vi "ClampingTargetDetect.vi"(0 "Image Src":T2) -> (14 "Image Out":T2(plugin-control), 15 "deltax":dbl, 16 "theta":dbl, 17 "distance":dbl, 19 "error out":errorcluster)   [LabVIEW 2011]
uses:
  <vilib>/vision/Image Controls.llb/IMAQ Image.ctl
  <vilib>/vision/Pattern Matching.llb/IMAQ Curve Parameters.ctl
  <vilib>/vision/NI_Vision_Development_Module.lvlib
panel:
  in  "Vertical":T1 {"Rotation" format="%.2f"; "Left" scale=0.0..1024.0; "Right" scale=0.0..1024.0}
  out "deltay":dbl
  in  "d0":dbl=115.0
  in  "p0":dbl=63.0
  in  "thresh":dbl=300.0
  in  "Horizontal":T1 {"Rotation" format="%.2f"; "Left" scale=0.0..1024.0; "Right" scale=0.0..1024.0}
  out "Clamp Points 2":T3
  out "Clamp Points":T3
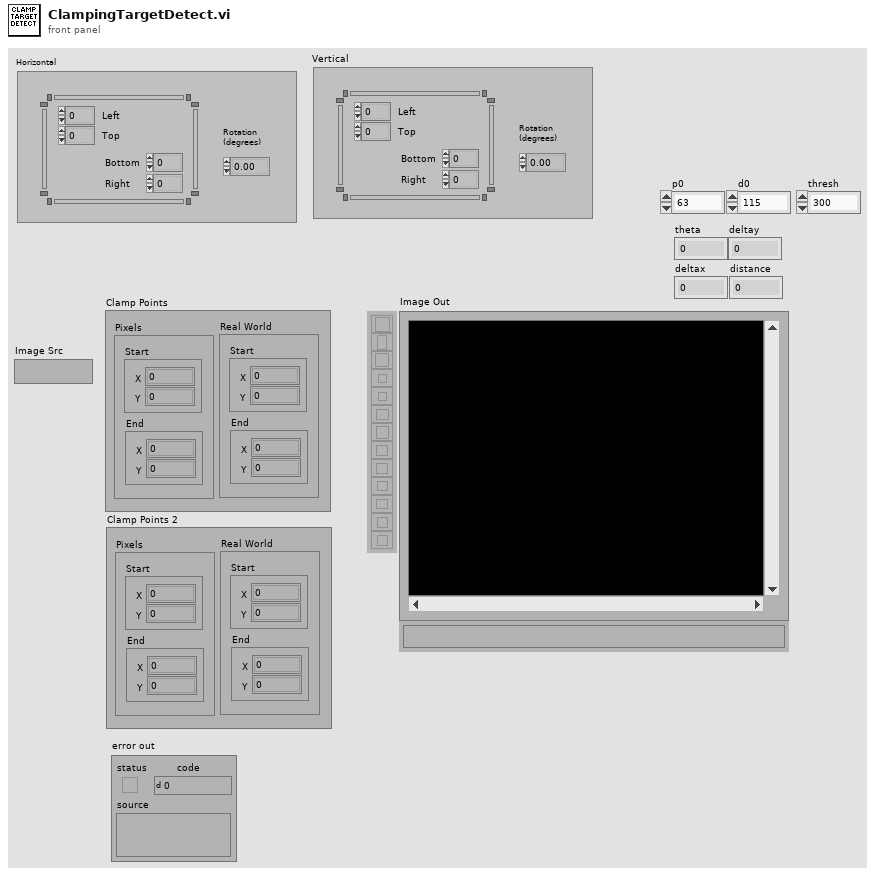
[diagram p1: front panel]
types:
  T1 = typedef "IMAQ Rectangle" = cluster{"Left":i32, "Top":i32, "Right":i32, "Bottom":i32, "Rotation":dbl}
  T2 = typedef "IMAQ Image.ctl" = refnum<image>
  T3 = cluster{"Pixels ":cluster{"Start":cluster{"X":dbl, "Y":dbl}, "End":cluster{"X":dbl, "Y":dbl}}, "Real World":cluster{"Start":cluster{"X":dbl, "Y":dbl}, "End":cluster{"X":dbl, "Y":dbl}}}
  T4 = cluster{"Angle Range (+/-)":dbl, "Edge Polarity":cluster{"Start":u32, "End":u32}}
  T5 = typedef "IMAQ Curve Parameters.ctl" = cluster{"Extraction Mode":u32, "Edge Threshold":i32, "Edge Filter Size":u32, "Min Length":i32, "Row Search Step Size":i32, "Col Search Step Size":i32, "Max Endpoint Gap":i32, "Closed":bool, "Subpixel":bool}
  T6 = cluster{"Show Search Area":bool, "Show Curves":bool, "Show Clamp Locations":bool, "Show Result":bool, "Search Area Color":u32, "Curves Color":u32, "Clamp Locations Color":u32, "Result Color":u32, "Overlay Group Name":string}
  T7 = cluster{"histogram":u32[], "Minimal Value":sgl, "Maximal Value":sgl, "Starting Value":sgl, "Interval Width":sgl, "Mean Value":sgl, "Standard  Variation":sgl, "Area (pixels)":i32}
  T8 = typedef "Image Type" = u32
  T9 = typedef "ROI Descriptor" = cluster{"Global Rectangle":i32[], "Contours":cluster{"ID":enum32{"External", "Internal"}, "Type":u32, "Coordinates":i32[]}[]}
  T10 = cluster{"Distance (Pixels)":dbl, "Distance (Real World)":dbl, "Angle (Absolute)":dbl, "Angle (Relative)":dbl}
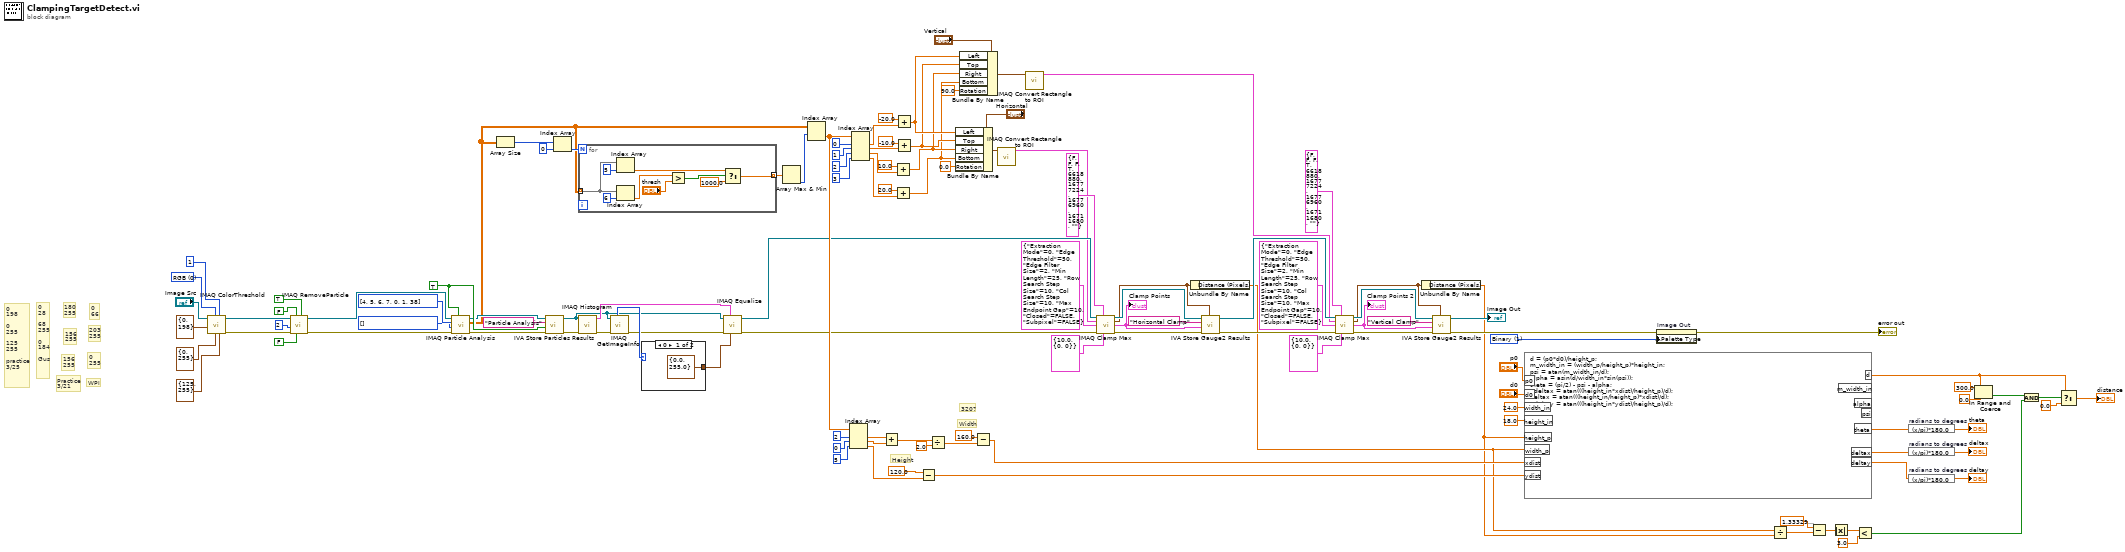
[diagram p0: block diagram]
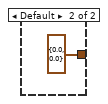
[diagram p2: hidden frame]
diagram:
  w82 = i32[] [] items=["Center of Mass X", "Center of Mass Y", "First Pixel X", "First Pixel Y", "Bounding Rect Left", "Bounding Rect Top", "Bounding Rect Right", "Bounding Rect Bottom", "Max Feret Diameter Start X", "Max Feret Diameter Start Y", "Max Feret Diameter End X", "Max Feret Diameter End Y", "Max Horiz. Segment Length Left", "Max Horiz. Segment Length Right", "Max Horiz. Segment Length Row", "-", "Bounding Rect Width", "Bounding Rect Height", "Bounding Rect Diagonal", "Perimeter", "Convex Hull Perimeter", "Holes' Perimeter", "Max Feret Diameter", "Equivalent Ellipse Major Axis", "Equivalent Ellipse Minor Axis", "Equivalent Ellipse Minor Axis (Feret)", "Equivalent Rect Long Side", "Equivalent Rect Short Side", "Equivalent Rect Diagonal", "Equivalent Rect Short Side (Feret)", "Average Horiz. Segment Length", "Average Vert. Segment Length", "Hydraulic Radius", "Waddel Disk Diameter", "-", "Area", "Holes' Area", "Particle & Holes' Area", "Convex Hull Area", "Image Area", "-", "Number of Holes", "Number of Horiz. Segments", "Number of Vert. Segments", "-", "Orientation", "Max Feret Diameter Orientation", "-", "% Area/Image Area", "% Area/(Particle & Holes' Area)", "Ratio of Equivalent Ellipse Axes", "Ratio of Equivalent Rect Sides", "-", "Elongation Factor", "Compactness Factor", "Heywood Circularity Factor", "Type Factor", "-", "Sum X", "Sum Y", "Sum XX", "Sum XY", "Sum YY", "Sum XXX", "Sum XXY", "Sum XYY", "Sum YYY", "-", "Moment of Inertia XX", "Moment of Inertia XY", "Moment of Inertia YY", "Moment of Inertia XXX", "Moment of Inertia XXY", "Moment of Inertia XYY", "Moment of Inertia YYY", "Norm. Moment of Inertia XX", "Norm. Moment of Inertia XY", "Norm. Moment of Inertia YY", "Norm. Moment of Inertia XXX", "Norm. Moment of Inertia XXY", "Norm. Moment of Inertia XYY", "Norm. Moment of Inertia YYY", "Hu Moment 1", "Hu Moment 2", "Hu Moment 3", "Hu Moment 4", "Hu Moment 5", "Hu Moment 6", "Hu Moment 7"] ("Real-World Measurements")
  w83 = i32[] [4, 5, 6, 7, 0, 1, 38] items=["Center of Mass X", "Center of Mass Y", "First Pixel X", "First Pixel Y", "Bounding Rect Left", "Bounding Rect Top", "Bounding Rect Right", "Bounding Rect Bottom", "Max Feret Diameter Start X", "Max Feret Diameter Start Y", "Max Feret Diameter End X", "Max Feret Diameter End Y", "Max Horiz. Segment Length Left", "Max Horiz. Segment Length Right", "Max Horiz. Segment Length Row", "-", "Bounding Rect Width", "Bounding Rect Height", "Bounding Rect Diagonal", "Perimeter", "Convex Hull Perimeter", "Holes' Perimeter", "Max Feret Diameter", "Equivalent Ellipse Major Axis", "Equivalent Ellipse Minor Axis", "Equivalent Ellipse Minor Axis (Feret)", "Equivalent Rect Long Side", "Equivalent Rect Short Side", "Equivalent Rect Diagonal", "Equivalent Rect Short Side (Feret)", "Average Horiz. Segment Length", "Average Vert. Segment Length", "Hydraulic Radius", "Waddel Disk Diameter", "-", "Area", "Holes' Area", "Particle & Holes' Area", "Convex Hull Area", "Image Area", "-", "Number of Holes", "Number of Horiz. Segments", "Number of Vert. Segments", "-", "Orientation", "Max Feret Diameter Orientation", "-", "% Area/Image Area", "% Area/(Particle & Holes' Area)", "Ratio of Equivalent Ellipse Axes", "Ratio of Equivalent Rect Sides", "-", "Elongation Factor", "Compactness Factor", "Heywood Circularity Factor", "Type Factor", "-", "Sum X", "Sum Y", "Sum XX", "Sum XY", "Sum YY", "Sum XXX", "Sum XXY", "Sum XYY", "Sum YYY", "-", "Moment of Inertia XX", "Moment of Inertia XY", "Moment of Inertia YY", "Moment of Inertia XXX", "Moment of Inertia XXY", "Moment of Inertia XYY", "Moment of Inertia YYY", "Norm. Moment of Inertia XX", "Norm. Moment of Inertia XY", "Norm. Moment of Inertia YY", "Norm. Moment of Inertia XXX", "Norm. Moment of Inertia XXY", "Norm. Moment of Inertia XYY", "Norm. Moment of Inertia YYY", "Hu Moment 1", "Hu Moment 2", "Hu Moment 3", "Hu Moment 4", "Hu Moment 5", "Hu Moment 6", "Hu Moment 7"] ("Pixel Measurements")
  w81 = TRUE ("Connectivity 4/8 (8)")
  w86 = u32 1 items=["Grayscale", "Binary", "Gradient", "Rainbow", "Temperature", "User Defined"] ("Palette")
  w119 = u16 0 items=["RGB", "HSL", "HSV", "HSI"] ("Color Mode")
  # "320?"
  # "0\n198\n\n0\n255\n\n125\n255\n\npractice\n3/25"
  # "0\n28\n\n68\n255\n\n0\n184\n\nGus"
  # "Practice\n3/21"
  # "WPI"
  # "156\n255"
  # "156\n255"
  # "180\n255"
  # "0\n255"
  # "203\n255"
  # "0\n66"
  # "Width"
  # "Height"
  n1 = call "IMAQ ColorThreshold"("Blue or Luma or Val or Inten Range"=cluster{"Lower value":i32, "Upper value":i32} {"Lower value"=125, "Upper value"=255}, "Replace Value"=1, "Green or Sat Range"=cluster{"Lower value":i32, "Upper value":i32} {"Lower value"=0, "Upper value"=255}, "Color Mode"=w119, "Red or Hue Range"=cluster{"Lower value":i32, "Upper value":i32} {"Lower value"=0, "Upper value"=198}, "Image Src"="Image Src") -> ("error out"=w115:errorcluster, "Image Dst Out"=w110:T2)  [unwired: 2 in, 2 out]
  n2 = call "IMAQ RemoveParticle"("Connectivity 4/8 (8)"=TRUE, "Low Pass/High Pass (Low)"=FALSE, "Square/Hexa (Square)"=FALSE, "error in (no error)"=w115, "Number of Erosion"=2, "Image Src"=w110) -> ("error out"=w43:errorcluster, "Image Dst Out"=w44:T2)  [unwired: 1 in, 3 out]
  n3 = call "IMAQ Particle Analysis"("Connectivity 4/8 (8)"=w81, "error in (no error)"=w43, "Real-World Measurements"=w82, "Pixel Measurements"=w83, "Image"=w44) -> ("error out"=w78:errorcluster, "Particle Measurements (Pixels)"=w56:dbl[][], "Image Out (duplicate)"=w80:T2)  [unwired: 4 out]
  n4 = Array Size(array=w56) -> (size(s)=w62:i32[])
  n5 = call <vilib>:"IVA Store Particles Results.vi"("error in (no error)"=w78, "Connectivity 4/8 (8)"=w81, "Step Name"="Particle Analysis", "Image in"=w80) -> ("error out"=w26:errorcluster, "Image dup"=w25:T2)  [unwired: 6 out]
  n6 = Index Array(array=w62, index=0) -> (element=w60:i32)
  n7 = for {
    N: w60 -> [_]
    tunnel: w56 -> [w127] mode=indexing
    tunnel: [w121] -> w55 mode=indexing
    n8 = Index Array(array=w127, index=5) -> (element=w123:dbl)
    n9 = Index Array(array=w127, index=6) -> (element=w126:dbl)
    n10 = Greater?(x=w126, y="thresh") -> (0:w124:bool)
    n11 = Select(t=w123, s=w124, f=1000.0) -> (s? t:f=w121:dbl)
  }
  n12 = call "IMAQ Histogram"("error in (no error)"=w26, "Image"=w25) -> ("error out"=w107:errorcluster, "Histogram Report"=w109:T7)  [unwired: 3 in, 5 out]
  n13 = call "IMAQ GetImageInfo"("error in (no error)"=w107, "Image"=w25) -> ("error out"=w106:errorcluster, "Image Type"=w108:T8)  [unwired: 8 out]
  n14 = case shown="0" w108 {
    tunnel: [cluster{"Minimum":sgl, "Maximum":sgl} {"Minimum"=0.0, "Maximum"=255.0} ("Range") cluster{"Minimum":sgl, "Maximum":sgl} {"Minimum"=0.0, "Maximum"=0.0} ("Range")] -> w105
    frame 0 {
    }
    frame Default {
    }
  }
  n15 = call "IMAQ Equalize"("Range"=w105, "Histogram Report"=w109, "error in (no error)"=w106, "Image Src"=w25) -> ("error out"=w45:errorcluster, "Image Dst Out"=w46:T2)  [unwired: 2 in, 4 out]
  n16 = Array Max & Min(array=w55) -> (min index (indices)=w59:i32)  [unwired: 3 out]
  n17 = Index Array(array=w56, index (row)=w59) -> (element=w65:dbl[])  [unwired: 1 in]
  n18 = Index Array(array=w65, index #1=2 ("index"), index #2=0 ("index"), index #3=5 ("index")) -> (element #1=w52:dbl, element #2=w51:dbl, element #3=w53:dbl)
  n19 = Index Array(array=w65, index #1=0 ("index"), index #2=1 ("index"), index #3=2 ("index"), index #4=3 ("index")) -> (element #1=w67:dbl, element #2=w72:dbl, element #3=w73:dbl, element #4=w71:dbl)
  n20 = Add(x=w52, y=w51) -> (x+y=w50:dbl)
  n21 = Add(x=10.0, y=w73) -> (x+y=w21:dbl)
  n22 = Add(x=20.0, y=w71) -> (x+y=w20:dbl)
  n23 = Add(x=-20.0 ("y"), y=w67) -> (x+y=w23:dbl)
  n24 = Add(x=-10.0, y=w72) -> (x+y=w22:dbl)
  n25 = Subtract(x=120.0, y=w53) -> (x-y=w31:dbl)
  n26 = Divide(x=w50, y=2.0) -> (x/y=w48:dbl)
  n27 = Bundle By Name(cluster="Horizontal", "Left"=w23, "Top"=w22, "Right"=w21, "Bottom"=w20, "Rotation"=0.0) -> (w42:T1)
  n28 = Bundle By Name(cluster="Vertical", "Left"=w23, "Top"=w22, "Right"=w21, "Bottom"=w20, "Rotation"=90.0) -> (w17:T1)
  n29 = Subtract(x=160.0, y=w48) -> (x-y=w30:dbl)
  n30 = call "IMAQ Convert Rectangle to ROI"("Rectangle"=w42) -> ("ROI Descriptor"=w41:T9)  [unwired: 8 in, 1 out]
  n31 = call "IMAQ Convert Rectangle to ROI"("Rectangle"=w17) -> ("ROI Descriptor"=w16:T9)  [unwired: 8 in, 1 out]
  n32 = call "IMAQ Clamp Max"("Source Image"=w46, "Overlay Settings"=T6 {"Show Search Area"=FALSE, "Show Curves"=FALSE, "Show Clamp Locations"=FALSE, "Show Result"=TRUE, "Search Area Color"=6618880, "Curves Color"=16777224, "Clamp Locations Color"=16776960, "Result Color"=16711680, "Overlay Group Name"=""}, "ROI Descriptor"=w41, "Curve Extraction Settings"=T5 {"Extraction Mode"=0, "Edge Threshold"=50, "Edge Filter Size"=2, "Min Length"=25, "Row Search Step Size"=10, "Col Search Step Size"=10, "Max Endpoint Gap"=10, "Closed"=FALSE, "Subpixel"=FALSE}, "error in (no error)"=w45, "Clamp Settings"=T4 {"Angle Range (+/-)"=10.0, "Edge Polarity"={"Start"=0, "End"=0}}) -> ("Image Out"=w103:T2, "Clamp Results"=w40:T10, "Clamp Points"=w97:T3, "error out"=w104:errorcluster)  [unwired: 1 in, 5 out]
  "Clamp Points" <- w97
  n33 = Unbundle By Name(w40) -> ("Distance (Pixels)"=w10:dbl)
  n34 = call <vilib>:"IVA Store Gauge2 Results.vi"("Clamp Results"=w40, "error in (no error)"=w104, "Clamp Points"=w97, "Step Name"="Horizontal Clamp", "Image in"=w103) -> ("error out"=w102:errorcluster, "Image Out"=w95:T2)  [unwired: 5 out]
  n35 = call "IMAQ Clamp Max"("Source Image"=w95, "Overlay Settings"=T6 {"Show Search Area"=FALSE, "Show Curves"=FALSE, "Show Clamp Locations"=FALSE, "Show Result"=TRUE, "Search Area Color"=6618880, "Curves Color"=16777224, "Clamp Locations Color"=16776960, "Result Color"=16711680, "Overlay Group Name"=""}, "ROI Descriptor"=w16, "Curve Extraction Settings"=T5 {"Extraction Mode"=0, "Edge Threshold"=50, "Edge Filter Size"=2, "Min Length"=25, "Row Search Step Size"=10, "Col Search Step Size"=10, "Max Endpoint Gap"=10, "Closed"=FALSE, "Subpixel"=FALSE}, "error in (no error)"=w102, "Clamp Settings"=T4 {"Angle Range (+/-)"=10.0, "Edge Polarity"={"Start"=0, "End"=0}}) -> ("Image Out"=w94:T2, "Clamp Results"=w39:T10, "Clamp Points"=w88:T3, "error out"=w96:errorcluster)  [unwired: 1 in, 5 out]
  "Clamp Points 2" <- w88
  n36 = Unbundle By Name(w39) -> ("Distance (Pixels)"=w9:dbl)
  n37 = call <vilib>:"IVA Store Gauge2 Results.vi"("Clamp Results"=w39, "error in (no error)"=w96, "Clamp Points"=w88, "Step Name"="Vertical Clamp", "Image in"=w94) -> ("error out"=w93:errorcluster, "Image Out"=→"Image Out":T2)  [unwired: 5 out]
  n38 = formula code="d = (p0*d0)/height_p;\nm_width_in = (width_p/height_p)*height_in;\npsi = atan(m_width_in/d);\nalpha = asin(d/width_in*sin(psi));\ntheta = (pi/2) - psi - alpha;\n//deltax = atan(((height_in*xdist)/height_p)/d);\ndeltax = atan(((height_in/height_p)*xdist)/d);\n//deltay = atan(((height_in*ydist)/height_p)/d);"("p0"="p0", "d0"="d0", "width_in"=24.0 ("input variable"), "height_in"=18.0 ("input variable"), "height_p"=w9, "width_p"=w10, "xdist"=w30, "ydist"=w31) -> ("d"=w3:dbl, "theta"=w34:dbl, "deltax"=w33:dbl, "deltay"=w32:dbl)  [unwired: 3 out]
  n39 = property on="Image Out" class="ImageControl"(error in=w93, "Palette:Palette Type"=w86) -> (error out=→"error out":errorcluster)  [unwired: 1 in, 1 out]
  n40 = Divide(x=w10, y=w9) -> (x/y=w15:dbl)
  n41 = Subtract(x=sgl 1.3333, y=w15) -> (x-y=w13:dbl)
  n42 = Absolute Value(x=w13) -> (abs(x)=w12:dbl)
  n43 = Less?(x=w12, y=sgl 3.0) -> (x < y?=w1:bool)
  n44 = expression code="(x/pi)*180.0" "radians to degrees"(w34) -> (→"theta":dbl)
  n45 = expression code="(x/pi)*180.0" "radians to degrees"(w33) -> (→"deltax":dbl)
  n46 = expression code="(x/pi)*180.0" "radians to degrees"(w32) -> (→"deltay":dbl)
  n47 = In Range and Coerce(upper limit=300.0, x=w3, lower limit=0.0) -> (In Range?=w2:bool)  [unwired: 1 out]
  n48 = And(x=w2, y=w1) -> (x .and. y?=w5:bool)
  n49 = Select(t=w3, s=w5, f=0.0) -> (s? t:f=→"distance":dbl)
